vi "Create_conn.vi"(0 "VISA resourceINPUT":refnum<visa-resource-name>) -> (1 "error out":errorcluster, 2 "VISA resource name out":refnum<visa-resource-name>)   [LabVIEW 2011]
uses:
  <vilib>/Instr/_visa.llb/VISA Configure Serial Port (Instr).vi
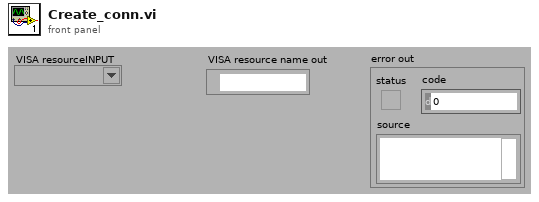
[diagram p1: front panel]
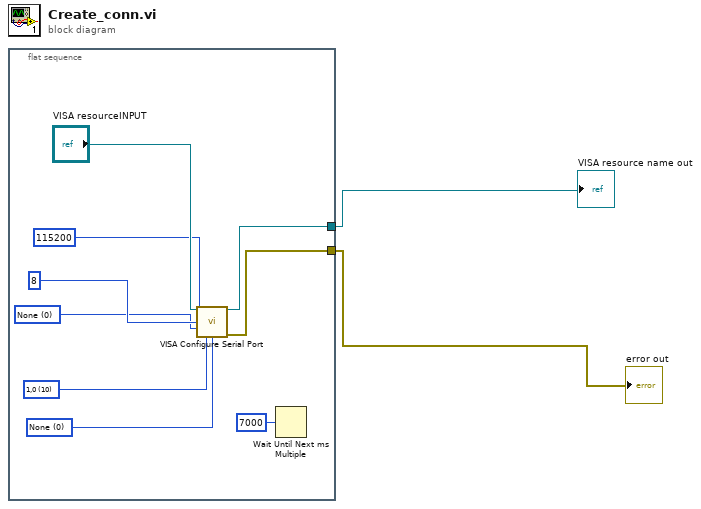
[diagram p0: block diagram]
diagram:
  n1 = flat-sequence {
    tunnel: [w5] -> w2
    tunnel: [w4] -> w1
    frame #0 {
      w6 = u16 0 items=["None"=0, "XON/XOFF"=1, "RTS/CTS"=2, "DTR/DSR"=4] ("Control de flujo")
      w7 = u16 10 items=["1,0"=10, "1,5"=15, "2,0"=20] ("Bits de paridad")
      w8 = u16 0 items=["None", "Odd", "Even", "Mark", "Space"] ("Paridad")
      n2 = call-poly "VISA Configure Serial Port"("VISA resource name"="VISA resourceINPUT", "baud rate (9600)"=u32 115200 ("Baudios"), "data bits (8)"=u16 8 ("Bits de datos"), "parity (0:none)"=w8, "stop bits (10: 1 bit)"=w7, "flow control (0:none)"=w6) -> ("VISA resource name out"=w4:refnum<visa-resource-name>, "error out"=w5:errorcluster)  [unwired: 8 in]
      n3 = Wait Until Next ms Multiple(millisecond multiple=u32 7000) -> ()  [unwired: 1 out]
    }
  }
  "error out" <- w2
  "VISA resource name out" <- w1
